vi "Create Signal Dictionaries.vi"(8 "error In":errorcluster, 10 "Raw Data":string[][](array[string])) -> (0 "Error Out":errorcluster, 2 "Parameter Array Out":refnum<class "String Database.lvclass">[](array[class]))   [LabVIEW 2016, in "TSF Parser.lvlib" / "TSF Parser.lvclass"]
uses:
  TSF Parser.lvclass
  Plugins/String Database.lvlibp/String Database.lvclass
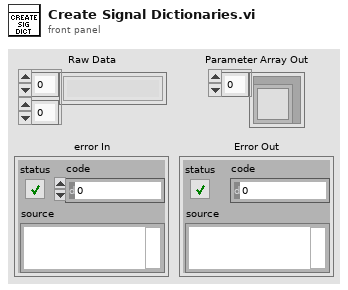
[diagram p1: front panel]
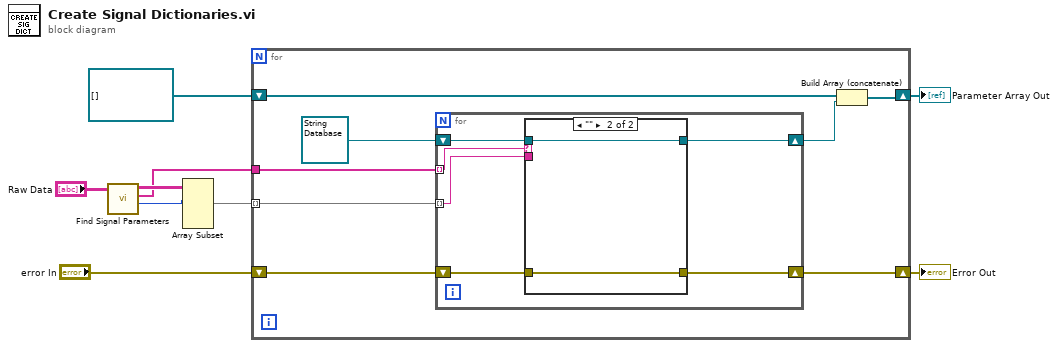
[diagram p0: block diagram]
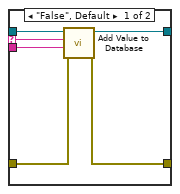
[diagram p2: hidden frame]
diagram:
  n1 = call "Find Signal Parameters.vi"("Worksheet Data"="Raw Data") -> ("Signal Parameter Row Index"=w7:i32, "Signal Parameters"=w4:string[], "Worksheet Data Out"=w8:string[][])  [unwired: 8 in]
  n2 = Array Subset(array=w8, index (row)=w7) -> (w5:string[][])  [unwired: 3 in]
  n3 = for {
    shift-right: [w10] -> w2
    shift-left: refnum<class "String Database.lvclass">[] [] -> [w12]
    tunnel: w5 -> [w15] mode=indexing
    tunnel: w4 -> [w16]
    shift-right: [w14] -> w1
    shift-left: "error In" -> [w13]
    n4 = for {
      shift-right: [w22] -> w11
      shift-left: refnum<class "String Database.lvclass"> refnum ("String Database out") -> [w23]
      tunnel: w16 -> [w21] mode=indexing
      tunnel: w15 -> [w20] mode=indexing
      shift-right: [w19] -> w14
      shift-left: w13 -> [w18]
      n5 = case shown="\"\"" w21 {
        selector: w21 -> [w27 _]
        tunnel: w23 -> [w29 w31]
        tunnel: [w28 w31] -> w22
        tunnel: w20 -> [w26 _]
        tunnel: [w25 w30] -> w19
        tunnel: w18 -> [w24 w30]
        frame "False", Default {
          n6 = call "Add Value to Database.vi"("error in (no error)"=w24, "Entry Value"=w26, "Entry Name"=w27, "Dictionary In"=w29) -> ("error out"=w25:errorcluster, "Dictionary Out"=w28:refnum<class "String Database.lvclass">)  [unwired: 5 in, 1 out]
        }
        frame "" {
        }
      }
    }
    n7 = Build Array (concatenate)(w12, w11) -> (w10:refnum<class "String Database.lvclass">[])
  }
  "Parameter Array Out" <- w2
  "Error Out" <- w1
